vi "image queue to disk and to display queue_grMD.vi"() -> ()   [LabVIEW 2012]
doc: "SciScan 1.2 160622"
uses:
  <vilib>/Utility/VariantDataType/Type.ctl
  Custom Controls/file format type def.ctl
  GFG/GFGnumericGet.vi
  GFG/GFGfpRefGet.vi
  GFG/GFGbooleanGet.vi
  image & display/save images/save channels to raw bin files.vi
  image & display/save images/save channels to interleaved multi-tiff files.vi
  image & display/save images/save channels to separate multi-tiff files.vi
  image & display/save images/save channels to stacked multi-tiff files.vi
  image & display/save images/save channels to interleaved tiff series.vi
  image & display/save images/save channels to separate tiff series.vi
  image & display/save images/save channels to stacked tiff series.vi
  GFG/GFG library.lvlib
  <vilib>/Utility/VariantDataType/VariantType.lvlib
panel:
  out "VI is running":bool
  in  "Stop Button":bool
  out "error out 4":errorcluster
  out "error out 3":errorcluster
  out "error out 2":errorcluster
  out "# elements in image data queue":i32
  out "error out":errorcluster
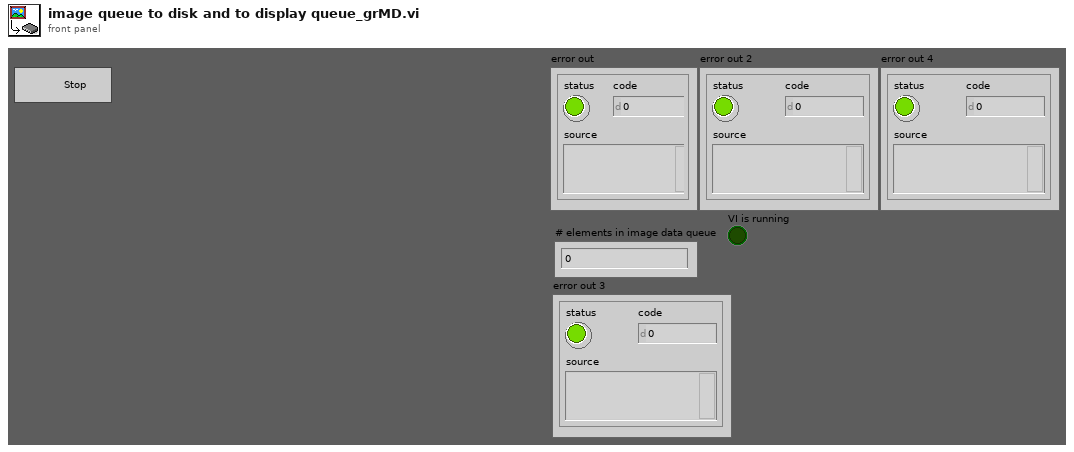
[diagram p1: front panel]
types:
  T1 = cluster{"Variable Name in":string, "Variant Out":variant}
  T2 = typedef "file format type def.ctl" = enum16{"16bit raw", "32bit raw", "16bit multi-tiff (interleave)", "16bit multi-tiff (separate)", "16bit multi-tiff (stacked)", "32bit multi-tiff (interleave)", "32bit multi-tiff (separate)", "32bit multi-tiff (stacked)", "16bit tiff series (interleave)", "16bit tiff series (separate)", "16bit tiff series (stacked)", "32bit tiff series (interleave)", "32bit tiff series (separate)", "32bit tiff series (stacked)"}
  T3 = enum8{"Enabled", "Disabled", "Disabled and Grayed Out"}
  T4 = cluster{"NewVal":bool, "Event Registration Refnum":refnum<event-registration>}
  T5 = cluster{"WaveformChartRef":refnum<vi>, "DigitalRef":refnum<vi>, "ArrayRef":refnum<vi>, "TabControlRef":refnum<vi>, "EnumRef":refnum<vi>, "RingRef":refnum<vi>, "BooleanRef":refnum<vi>, "KnobRef":refnum<vi>, "SlideRef":refnum<vi>, "PathRef":refnum<vi>, "StringRef":refnum<vi>, "ComboBox":refnum<vi>, "WaveformGraphRef":refnum<vi>}
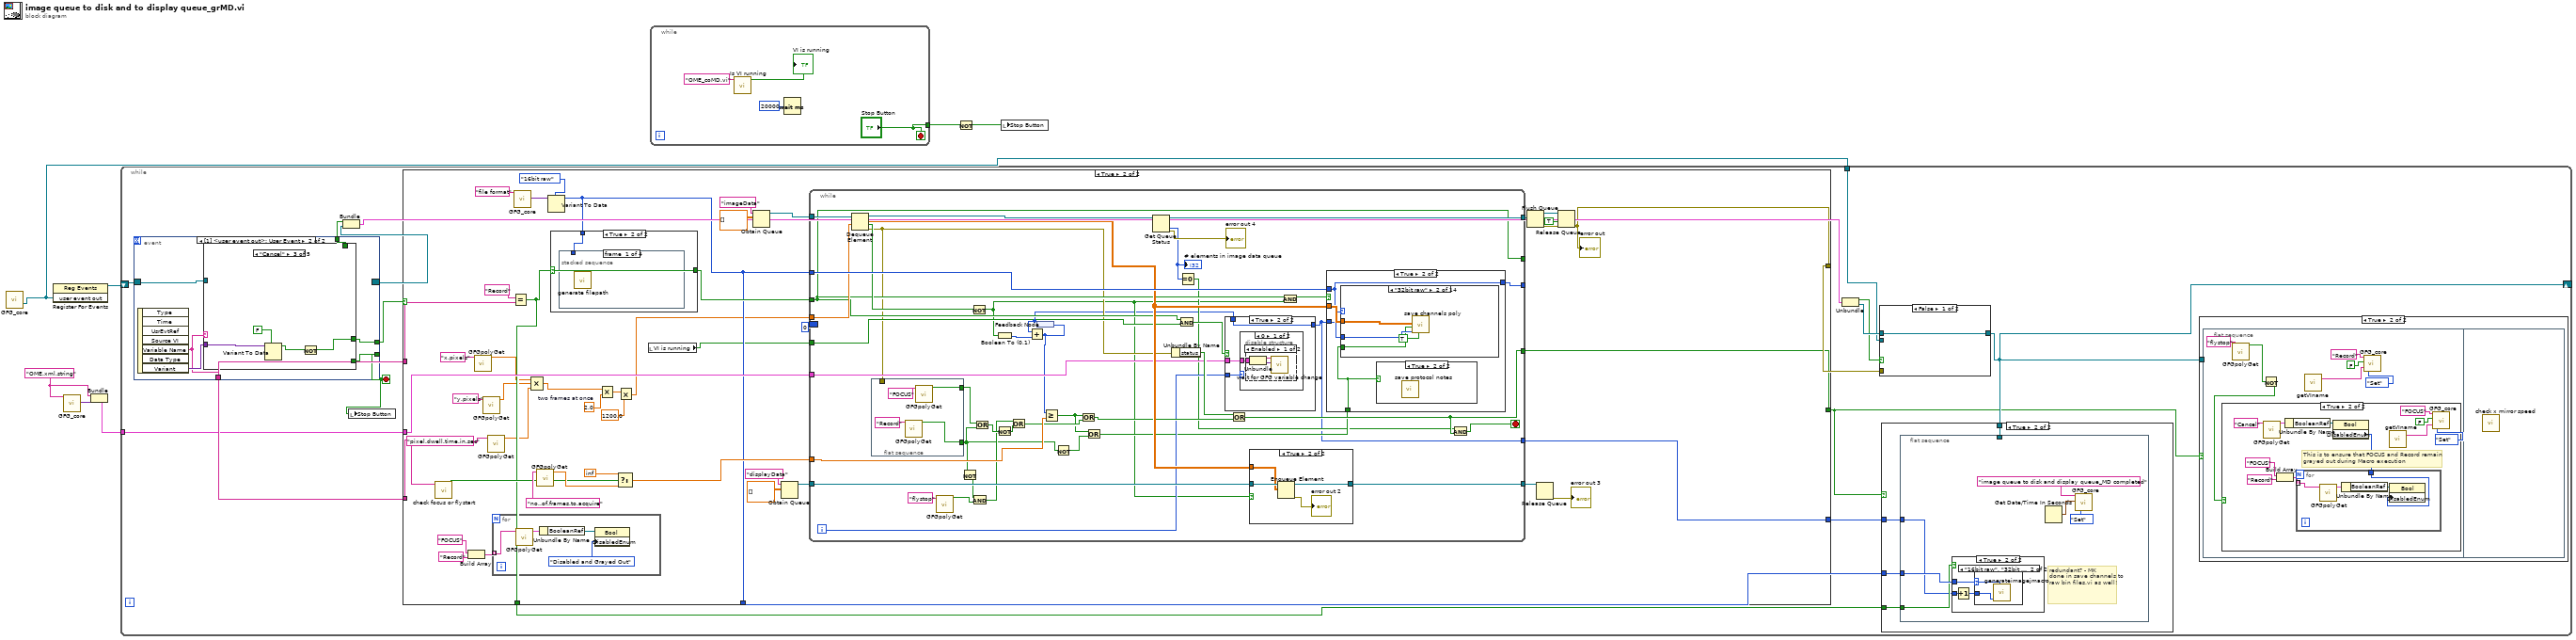
[diagram p0: block diagram]
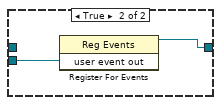
[diagram p7: hidden frame]
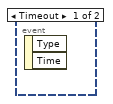
[diagram p8: hidden frame]
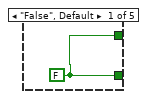
[diagram p9: hidden frame]
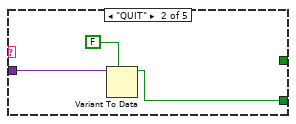
[diagram p10: hidden frame]
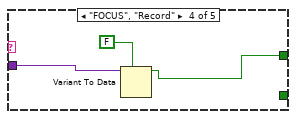
[diagram p11: hidden frame]
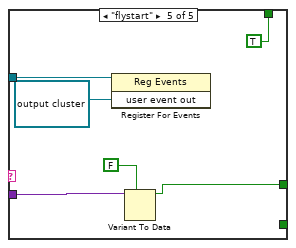
[diagram p12: hidden frame]
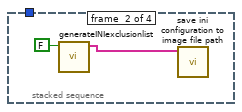
[diagram p15: hidden frame]
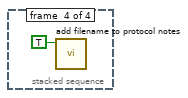
[diagram p17: hidden frame]
diagram:
  w4 = "OME.xml.string" ("Variable Name in")
  n1 = call "GFG_core.vi"() -> ("user event out"=w6:refnum<user-event>)  [unwired: 13 in, 6 out]
  n2 = register-events(w6) -> (reference out=w7:refnum<event-registration>)  [unwired: 2 in, 1 out]
  n3 = call "GFG_core.vi"("Variable Name in"=w4) -> ("Variant Out"=w3:variant)  [unwired: 12 in, 6 out]
  n4 = Bundle("Variable Name in"=w4, "Variant Out"=w3) -> (w5:T1)  [unwired: 1 in]
  n5 = while {
    tunnel: w6 -> [w16]
    shift-right: [w14] -> _
    shift-left: w7 -> [w23]
    tunnel: w5 -> [w12]
    stop <- w8 stop-if-true
    n6 = event shown="[1] <user event out>: User Event" {
      selector: w23 -> [_ w66]
      dyn-events: [_ _] -> w21
      timeout: _ -> [_ _]
      tunnel: [_ w70] -> w24
      tunnel: [_ w69] -> w8
      tunnel: [_ w67] -> w15
      tunnel: [_ w65] -> w22
      event Timeout {
        n7 = event-data() -> ()  [unwired: 1 in, 2 out]
      }
      event User Event {
        n8 = event-data() -> ("Variable Name"=w67:string, "Variant"=w68:variant)  [unwired: 1 in, 5 out]
        n9 = case shown="\"Cancel\"" w67 {
          tunnel: [w71 _ w75 w79 w85] -> w70
          tunnel: [w71 w72 _ _ _] -> w69
          tunnel: w68 -> [_ w74 w77 w80 w86]
          tunnel: w66 -> [_ _ _ _ w83]
          tunnel: [_ _ _ _ TRUE ("NewVal")] -> w65
          frame "False", Default {
            w71 = FALSE ("NewVal")
          }
          frame "QUIT" {
            n10 = Variant To Data(type=FALSE ("NewVal"), Variant=w74) -> (data=w72:bool)  [unwired: 1 in, 1 out]
          }
          frame "Cancel" {
            n11 = Variant To Data(type=FALSE ("NewVal"), Variant=w77) -> (data=w76:bool)  [unwired: 1 in, 1 out]
            n12 = Not(x=w76) -> (.not. x?=w75:bool)
          }
          frame "FOCUS", "Record" {
            n13 = Variant To Data(type=FALSE ("NewVal"), Variant=w80) -> (data=w79:bool)  [unwired: 1 in, 1 out]
          }
          frame "flystart" {
            n14 = register-events(reference=w83, refnum<user-event> refnum ("user event out")) -> ()  [unwired: 1 in, 2 out]
            n15 = Variant To Data(type=FALSE ("NewVal"), Variant=w86) -> (data=w85:bool)  [unwired: 1 in, 1 out]
          }
        }
      }
    }
    n16 = Bundle("NewVal"=w22, "Event Registration Refnum"=w21) -> (w19:T4)  [unwired: 1 in]
    n17 = local write "Stop Button"(w8) -> ()
    n18 = case shown="True" w24 {
      tunnel: w15 -> [_ w123]
      tunnel: [_ w116] -> w20
      tunnel: w15 -> [_ w111]
      tunnel: [_ w109] -> w13
      tunnel: w12 -> [_ w106]
      tunnel: [_ w105] -> w11
      tunnel: [_ w104] -> w10
      tunnel: [_ w103] -> w9
      frame False {
      }
      frame True {
        w99 = 2.0  # two frames at once
        n19 = call "check focus or flystart.vi"("GFG variable name"=w111) -> ("Focus or flystart?"=w110:bool)  [unwired: 10 in]
        n20 = Build Array("FOCUS" ("Variable Name in"), "Record" ("element")) -> (w102:string[])
        n21 = call-poly "GFGpolyGet.vi"("Variable Name in"="x.pixels") -> ("Numeric"=w92:dbl)  [unwired: 8 in, 2 out]
        n22 = call-poly "GFGpolyGet.vi"("Variable Name in"="y.pixels") -> ("Numeric"=w91:dbl)  [unwired: 8 in, 2 out]
        n23 = call-poly "GFGpolyGet.vi"("Variable Name in"="pixel.dwell.time.in.sec" ("Tag in")) -> ("Numeric"=w90:dbl)  [unwired: 8 in, 2 out]
        n24 = for {
          tunnel: w102 -> [w137] mode=indexing
          n25 = call-poly "GFGpolyGet.vi"("Variable Name in"=w137) -> ("output cluster"=w136:T5)  [unwired: 9 in, 1 out]
          n26 = Unbundle By Name(w136) -> ("BooleanRef"=w135:refnum<vi>)
          n27 = property class="Bool"(reference=w135, "DisabledEnum"=T3."Disabled and Grayed Out" ("Disabled")) -> ()  [unwired: 1 in, 2 out]
        }
        n28 = Equal?(x="Record", y=w123) -> (x = y?=w104:bool)
        n29 = call "GFG_core.vi"("Variable Name in"="file format") -> ("Variant Out"=w120:variant)  [unwired: 12 in, 6 out]
        n30 = Compound Arithmetic op=MULTIPLY(w92, w91, w90) -> (w89:dbl)
        n31 = call-poly "GFGpolyGet.vi"("Variable Name in"="no..of.frames.to.acquire" ("Tag in")) -> ("Numeric"=w113:dbl)  [unwired: 8 in, 2 out]
        n32 = Variant To Data(type=file_format_type_def."16bit raw" ("file format"), Variant=w120) -> (data=w105:T2)  [unwired: 1 in, 1 out]
        n33 = case shown="True" w104 {
          selector: w104 -> [w138 w140]
          tunnel: [w138 w140] -> w118
          tunnel: w105 -> [_ w139]
          frame False {
          }
          frame True {
            n34 = stacked-sequence {
              tunnel: w139 -> [_ _ _ _]
              frame #0 {
                n35 = call "generate filepath.vi"() -> ()  [unwired: 11 in, 1 out]
              }
              frame #1 {
                n36 = call "generateINIexclusionlist.vi"("T for reso, F for galvo"=FALSE) -> ("Array"=w142:string[])  [unwired: 10 in]
                n37 = call "save ini configuration to image file path.vi"("exclusion regexp array"=w142) -> ()  [unwired: 11 in]
              }
              frame #2 {
              }
              frame #3 {
                n38 = call "add filename to protocol notes.vi"("rec start/end (T is start)"=TRUE) -> ()  [unwired: 10 in, 1 out]
              }
            }
          }
        }
        n39 = Multiply(x=w89, y=w99) -> (x*y=w98:dbl)
        n40 = Select(t=inf, s=w110, f=w113) -> (s? t:f=w112:dbl)
        n41 = Multiply(x=w98, y=1200.0) -> (x*y=w96:dbl)
        n42 = local read "VI is running"() -> (w88:bool)
        n43 = Obtain Queue(name (unnamed)="imageData", element data type=dbl[][] [] ("y backward image")) -> (queue out=w124:refnum<queue>)  [unwired: 3 in, 2 out]
        n44 = Obtain Queue(name (unnamed)="displayData", element data type=dbl[][] [] ("y backward image")) -> (queue out=w131:refnum<queue>)  [unwired: 3 in, 2 out]
        n45 = while {
          tunnel: [w179] -> w129
          tunnel: w131 -> [w182]
          tunnel: [w185] -> w130
          tunnel: w112 -> [w183]
          tunnel: w96 -> [w174]
          tunnel: w124 -> [w181]
          tunnel: w118 -> [w159]
          tunnel: w105 -> [w178]
          tunnel: [w159] -> _
          tunnel: [w177] -> _
          tunnel: [w175] -> w109
          border: i16 0 -> [_]
          tunnel: w106 -> [w160]
          tunnel: w88 -> [w152]
          tunnel: [w144] -> w103
          i -> [w158]
          stop <- w150 stop-if-true
          n46 = Dequeue Element(queue=w181, timeout in ms (-1)=w174) -> (queue out=w180:refnum<queue>, element=w176:dbl[][], timed out?=w161:bool, error out=w151:errorcluster)  [unwired: 1 in]
          n47 = flat-sequence {
            tunnel: [w187] -> w171
            tunnel: [w186] -> w157
            tunnel: w151 -> [_]
            frame #0 {
              n48 = call-poly "GFGpolyGet.vi"("Variable Name in"="Record") -> ("Boolean Value OUT"=w186:bool)  [unwired: 9 in, 1 out]
              n49 = call-poly "GFGpolyGet.vi"("Variable Name in"="FOCUS") -> ("Boolean Value OUT"=w187:bool)  [unwired: 9 in, 1 out]
            }
          }
          n50 = call-poly "GFGpolyGet.vi"("Variable Name in"="flystop") -> ("Boolean Value OUT"=w166:bool)  [unwired: 9 in, 1 out]
          n51 = Not(x=w157) -> (.not. x?=w167:bool)
          n52 = Not(x=w161) -> (.not. x?=w147:bool)
          n53 = And(x=w167, y=w166) -> (x .and. y?=w165:bool)
          n54 = Or(x=w171, y=w157) -> (x .or. y?=w170:bool)
          n55 = Not(x=w170) -> (.not. x?=w169:bool)
          n56 = Boolean To (0,1)(Boolean=w147) -> (0, 1=w162:i16)
          n57 = Or(x=w165, y=w169) -> (x .or. y?=w163:bool)
          n58 = feedback #1() -> (w145:i16)
          n59 = Add(x=w145, y=w162) -> (x+y=w146:i16)
          n60 = feedback-in #1(w146) -> ()
          n61 = Greater Or Equal?(x=w146, y=w183) -> (x >= y?=w155:bool)
          n62 = Not(x=w157) -> (.not. x?=w156:bool)
          n63 = Or(x=w155, y=w163) -> (x .or. y?=w164:bool)
          n64 = Or(x=w155, y=w156) -> (x .or. y?=w154:bool)
          n65 = Get Queue Status(queue=w180) -> (queue out=w179:refnum<queue>, error out=→"error out 4":errorcluster, # elements in queue=w149:i32)  [unwired: 2 in, 5 out]
          "# elements in image data queue" <- w149
          n66 = Unbundle By Name(w151) -> ("status"=w184:bool)
          n67 = And(x=w159, y=w152) -> (x .and. y?=w153:bool)
          n68 = Equal To 0?(x=w149) -> (x = 0?=w148:bool)
          n69 = case shown="True" w153 {
            tunnel: w145 -> [w190 w191]
            tunnel: w160 -> [_ w193]
            tunnel: w158 -> [_ w192]
            tunnel: [w190 w191] -> w144
            frame False {
            }
            frame True {
              n70 = case shown="0" w192 {
                tunnel: w193 -> [w194 _]
                frame 0 {
                  n71 = disable-structure shown="Enabled" {
                    disable-tunnel: w194 -> [w197 _]
                    frame Enabled {
                      n72 = Unbundle(w197) -> ("Variable Name in"=w196:string, "Variant Out"=w195:variant)
                      n73 = call "wait for GFG variable change.vi"("Initialization Value"=w195, "Variable Name in"=w196) -> ()  [unwired: 9 in, 1 out]
                    }
                    frame Disabled {
                    }
                  }
                }
                frame 1, Default {
                }
              }
            }
          }
          n74 = Or(x=w184, y=w164) -> (x .or. y?=w175:bool)
          n75 = case shown="True" w147 {
            tunnel: [w198 w202] -> w185
            tunnel: w182 -> [w198 w201]
            tunnel: w176 -> [_ w200]
            frame False {
            }
            frame True {
              n76 = Enqueue Element(queue=w201, element=w200) -> (queue out=w202:refnum<queue>, error out=→"error out 2":errorcluster)  [unwired: 2 in, 1 out]
            }
          }
          n77 = And(x=w159, y=w147) -> (x .and. y?=w173:bool)
          n78 = case shown="True" w173 {
            tunnel: w144 -> [_ w206]
            tunnel: w178 -> [w203 w205]
            tunnel: w176 -> [_ w207]
            tunnel: [w203 w205] -> w177
            tunnel: w154 -> [_ w204]
            frame False {
            }
            frame True {
              n79 = case shown="\"32bit raw\"" w205 {
                tunnel: w207 -> [w210 w216 w220 w226 w232 w239 w242 w245 w247 w253 w259 w266 w269 w272]
                tunnel: w206 -> [w214 w218 w224 w230 w236 w238 w241 w244 w251 w257 w263 w265 w268 w271]
                tunnel: w204 -> [w213 w217 w223 w229 w235 w237 w240 w243 w250 w256 w262 w264 w267 w270]
                frame "16bit raw" {
                  n80 = Add(x=i16 32767, y=w210) -> (x+y=w212:dbl[][])
                  n81 = To Unsigned Word Integer(number=w212) -> (unsigned 16bit integer=w209:u16[][])
                  n82 = call-poly "save channels poly.vi"("T:galvo F:resonant default:T"=TRUE, "frame number in"=w214, "last frame"=w213, "image data in (U16)"=w209) -> ()  [unwired: 8 in]
                }
                frame "32bit raw" {
                  n83 = call-poly "save channels poly.vi"("T:galvo F:resonant default:T"=TRUE, "frame number in"=w218, "last frame"=w217, "image data in (SGL)"=w216) -> ()  [unwired: 8 in]
                }
                frame "16bit multi-tiff (interleave)" {
                  n84 = Add(x=i16 32767, y=w220) -> (x+y=w222:dbl[][])
                  n85 = To Unsigned Word Integer(number=w222) -> (unsigned 16bit integer=w219:u16[][])
                  n86 = call-poly "save channels poly.vi"("frame number in"=w224, "last frame"=w223, "image data in"=w219) -> ()  [unwired: 9 in]
                }
                frame "16bit multi-tiff (separate)" {
                  n87 = Add(x=i16 32767, y=w226) -> (x+y=w228:dbl[][])
                  n88 = To Unsigned Word Integer(number=w228) -> (unsigned 16bit integer=w225:u16[][])
                  n89 = call-poly "save channels poly.vi"("frame number in"=w230, "last frame"=w229, "image data in"=w225) -> ()  [unwired: 9 in]
                }
                frame "16bit multi-tiff (stacked)" {
                  n90 = Add(x=i16 32767, y=w232) -> (x+y=w234:dbl[][])
                  n91 = To Unsigned Word Integer(number=w234) -> (unsigned 16bit integer=w231:u16[][])
                  n92 = call-poly "save channels poly.vi"("frame number in"=w236, "last frame"=w235, "image data in"=w231) -> ()  [unwired: 9 in]
                }
                frame "32bit multi-tiff (interleave)" {
                  n93 = call-poly "save channels poly.vi"("frame number in"=w238, "last frame"=w237, "image data in"=w239) -> ()  [unwired: 9 in]
                }
                frame "32bit multi-tiff (separate)" {
                  n94 = call-poly "save channels poly.vi"("frame number in"=w241, "last frame"=w240, "image data in"=w242) -> ()  [unwired: 9 in]
                }
                frame "32bit multi-tiff (stacked)" {
                  n95 = call-poly "save channels poly.vi"("frame number in"=w244, "last frame"=w243, "image data in"=w245) -> ()  [unwired: 9 in]
                }
                frame "16bit tiff series (interleave)" {
                  n96 = Add(x=i16 32767, y=w247) -> (x+y=w249:dbl[][])
                  n97 = To Unsigned Word Integer(number=w249) -> (unsigned 16bit integer=w246:u16[][])
                  n98 = call-poly "save channels poly.vi"("frame number in"=w251, "last frame"=w250, "image data in"=w246) -> ()  [unwired: 9 in]
                }
                frame "16bit tiff series (separate)" {
                  n99 = Add(x=i16 32767, y=w253) -> (x+y=w255:dbl[][])
                  n100 = To Unsigned Word Integer(number=w255) -> (unsigned 16bit integer=w252:u16[][])
                  n101 = call-poly "save channels poly.vi"("frame number in"=w257, "last frame"=w256, "image data in"=w252) -> ()  [unwired: 9 in]
                }
                frame "16bit tiff series (stacked)" {
                  n102 = Add(x=i16 32767, y=w259) -> (x+y=w261:dbl[][])
                  n103 = To Unsigned Word Integer(number=w261) -> (unsigned 16bit integer=w258:u16[][])
                  n104 = call-poly "save channels poly.vi"("frame number in"=w263, "last frame"=w262, "image data in"=w258) -> ()  [unwired: 9 in]
                }
                frame "32bit tiff series (interleave)" {
                  n105 = call-poly "save channels poly.vi"("frame number in"=w265, "last frame"=w264, "image data in"=w266) -> ()  [unwired: 9 in]
                }
                frame "32bit tiff series (separate)" {
                  n106 = call-poly "save channels poly.vi"("frame number in"=w268, "last frame"=w267, "image data in"=w269) -> ()  [unwired: 9 in]
                }
                frame "32bit tiff series (stacked)" {
                  n107 = call-poly "save channels poly.vi"("frame number in"=w271, "last frame"=w270, "image data in"=w272) -> ()  [unwired: 9 in]
                }
              }
              n108 = case shown="True" w204 {
                frame False {
                }
                frame True {
                  n109 = call "save protocol notes.vi"() -> ()  [unwired: 12 in]
                }
              }
            }
          }
          n110 = And(x=w148, y=w175) -> (x .and. y?=w150:bool)
        }
        n111 = Flush Queue(queue=w129) -> (queue out=w128:refnum<queue>, error out=w127:errorcluster)  [unwired: 1 in, 1 out]
        n112 = Release Queue(queue=w130) -> (error out=→"error out 3":errorcluster)  [unwired: 2 in, 2 out]
        n113 = Release Queue(queue=w128, force destroy? (F)=TRUE, error in (no error)=w127) -> (error out=w116:errorcluster)  [unwired: 2 out]
        "error out" <- w116
      }
    }
    n114 = Unbundle(w19) -> ("NewVal"=w17:bool, "Event Registration Refnum"=w18:refnum<event-registration>)
    n115 = case shown="False" w17 {
      tunnel: [w62 w64] -> w14
      tunnel: w16 -> [_ w63]
      tunnel: w20 -> [_ _]
      tunnel: w18 -> [w62 _]
      frame False {
      }
      frame True {
        n116 = register-events(w63) -> (reference out=w64:refnum<event-registration>)  [unwired: 2 in, 1 out]
      }
    }
    n117 = case shown="True" w13 {
      tunnel: w14 -> [_ w50]
      tunnel: w11 -> [_ w49]
      tunnel: w10 -> [_ w48]
      tunnel: w9 -> [_ w47]
      frame False {
      }
      frame True {
        n118 = flat-sequence {
          tunnel: w50 -> [_]
          tunnel: w49 -> [w53]
          tunnel: w48 -> [w52]
          tunnel: w47 -> [w51]
          frame #0 {
            # "redundant? - MK\ndone in save channels to raw bin files.vi as well!"
            n119 = case shown="True" w52 {
              tunnel: w53 -> [_ w59]
              tunnel: w51 -> [_ w58]
              frame False {
              }
              frame True {
                n120 = Increment(x=w58) -> (x+1=w57:i16)
                n121 = case shown="\"16bit raw\", \"32bit raw\"" w59 {
                  selector: w59 -> [_ w61]
                  tunnel: w57 -> [_ w60]
                  frame Default {
                  }
                  frame "16bit raw", "32bit raw" {
                    n122 = call "generateimagejmacro.vi"("file format"=w61, "number of recorded frames"=w60) -> ()  [unwired: 10 in]
                  }
                }
              }
            }
            n123 = Get Date/Time In Seconds() -> (seconds since 1Jan1904=w54:timestamp)
            n124 = call "GFG_core.vi"("Variable Name in"="image queue to disk and display queue_MD completed", "Variant in"=w54, "Action"=enum16{"Init", "Set", "Get"}."Set") -> ()  [unwired: 10 in, 7 out]
          }
        }
      }
    }
    n125 = case shown="True" w13 {
      tunnel: w14 -> [_ _]
      frame False {
      }
      frame True {
        n126 = flat-sequence {
          frame #0 {
            n127 = call-poly "GFGpolyGet.vi"("Variable Name in"="flystop") -> ("Boolean Value OUT"=w30:bool)  [unwired: 9 in, 1 out]
            n128 = Not(x=w30) -> (.not. x?=w31:bool)
            n129 = case shown="True" w31 {
              frame False {
              }
              frame True {
                # "This is to ensure that FOCUS and Record remain\ngrayed out during Macro execution"
                n130 = call-poly "GFGpolyGet.vi"("Variable Name in"="Cancel") -> ("output cluster"=w33:T5)  [unwired: 9 in, 1 out]
                n131 = Build Array("FOCUS" ("Variable Name in"), "Record" ("element")) -> (w38:string[])
                n132 = Unbundle By Name(w33) -> ("BooleanRef"=w34:refnum<vi>)
                n133 = property class="Bool"(reference=w34) -> ("DisabledEnum"=w35:T3)  [unwired: 1 in, 2 out]
                n134 = for {
                  tunnel: w38 -> [w46] mode=indexing
                  tunnel: w35 -> [w43]
                  n135 = call-poly "GFGpolyGet.vi"("Variable Name in"=w46) -> ("output cluster"=w45:T5)  [unwired: 9 in, 1 out]
                  n136 = Unbundle By Name(w45) -> ("BooleanRef"=w44:refnum<vi>)
                  n137 = property class="Bool"(reference=w44, "DisabledEnum"=w43) -> ()  [unwired: 1 in, 2 out]
                }
                n138 = call "getVIname.vi"() -> ("VI name"=w42:string)  [unwired: 19 in]
                n139 = call "GFG_core.vi"("Variable Name in"="FOCUS" ("Tag in"), "Variant in"=FALSE, "Source VI"=w42, "Action"=enum16{"Init", "Set", "Get"}."Set") -> ()  [unwired: 9 in, 7 out]
              }
            }
            n140 = call "getVIname.vi"() -> ("VI name"=w25:string)  [unwired: 19 in]
            n141 = call "GFG_core.vi"("Variable Name in"="Record" ("Tag in"), "Variant in"=FALSE, "Source VI"=w25, "Action"=enum16{"Init", "Set", "Get"}."Set") -> ()  [unwired: 9 in, 7 out]
          }
          frame #1 {
            n142 = call "check x mirror speed.vi"() -> ()  [unwired: 11 in, 1 out]
          }
        }
      }
    }
  }
  n143 = while {
    tunnel: ["Stop Button"] -> w2
    stop <- "Stop Button" stop-if-true
    n144 = call "Is VI running.vi"("VI name"="OME_coMD.vi") -> ("VI is running"=→"VI is running":bool)  [unwired: 9 in, 1 out]
    n145 = Wait (ms)(milliseconds to wait=u32 20000) -> ()  [unwired: 1 out]
  }
  n146 = Not(x=w2) -> (.not. x?=w1:bool)
  n147 = local write "Stop Button"(w1) -> ()
